vi "核查数据发送(子VI).vi"(8 "错误输入":errorcluster) -> (0 "错误输出":errorcluster)   [LabVIEW 2016, in "数据传输系统.lvlib"]
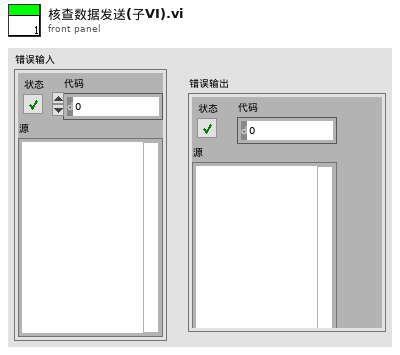
[diagram p1: front panel]
types:
  T1 = enum16{"质控数据", "操作日志", "仪器参数", "系统状态", "运行模式", "测量周期", "超标留样", "报警信息", "环境参数"}
  T2 = enum16{"空白测试", "跨度核查", "标样核查", "加标回收", "平行样", "集成干预"}
  T3 = cluster{"氨氮零点核查索引起始时间":string, "总磷零点核查索引起始时间":string, "总氮零点核查索引起始时间":string, "CODMn零点核查索引起始时间":string, "CODCr零点核查索引起始时间":string, "亚硝酸盐零点核查索引起始时间":string, "硫化物零点核查索引起始时间":string, "ORP零点核查索引起始时间":string}
  T4 = cluster{"数组[0]":string, "数组[1]":string, "数组[2]":string, "数组[3]":string, "数组[4]":string, "数组[5]":string, "数组[6]":string, "数组[7]":string}
  T5 = cluster{"PH":string[][], "CODCr":string[][], "氨氮":string[][], "CODMn":string[][], "总氮":string[][], "总磷":string[][], "电导率":string[][], "水温":string[][], "DO":string[][], "浊度":string[][], "叶绿素":string[][], "藻密度":string[][], "铜":string[][], "盐度":string[][], "水位":string[][], "流速":string[][], "瞬时流量":string[][], "累积流量":string[][], "亚硝酸盐":string[][], "硫化物":string[][], "ORP":string[][], "铅":string[][], "镉":string[][], "锌":string[][], "镍":string[][], "锰":string[][], "汞":string[][], "气温":string[][], "气压":string[][], "风速":string[][], "风向":string[][]}
  T6 = cluster{"氨氮跨度核查索引起始时间":string, "总磷跨度核查索引起始时间":string, "总氮跨度核查索引起始时间":string, "CODMn跨度核查索引起始时间":string, "CODCr跨度核查索引起始时间":string, "亚硝酸盐跨度核查索引起始时间":string, "硫化物跨度核查索引起始时间":string, "ORP跨度核查索引起始时间":string}
  T7 = cluster{"氨氮标样核查索引起始时间":string, "总磷标样核查索引起始时间":string, "总氮标样核查索引起始时间":string, "CODMn标样核查索引起始时间":string, "CODCr标样核查索引起始时间":string, "DO标样核查索引起始时间":string, "PH标样核查索引起始时间":string, "比电导率标样核查索引起始时间":string, "水温标样核查索引起始时间":string, "浊度标样核查索引起始时间":string, "叶绿素a标样核查索引起始时间":string, "藻密度标样核查索引起始时间":string, "亚硝酸盐标样核查索引起始时间":string, "硫化物标样核查索引起始时间":string, "ORP标样核查索引起始时间":string}
  T8 = cluster{"数组[0]":string, "数组[1]":string, "数组[2]":string, "数组[3]":string, "数组[4]":string, "数组[5]":string, "数组[6]":string, "数组[7]":string, "数组[8]":string, "数组[9]":string, "数组[10]":string, "数组[11]":string, "数组[12]":string, "数组[13]":string, "数组[14]":string}
  T9 = cluster{"氨氮加标回收索引起始时间":string, "总磷加标回收索引起始时间":string, "总氮加标回收索引起始时间":string, "CODMn加标回收索引起始时间":string, "CODCr加标回收索引起始时间":string}
  T10 = cluster{"[0]":string, "[1]":string, "[2]":string, "[3]":string, "[4]":string}
  T11 = cluster{"氨氮平行样索引起始时间":string, "总磷平行样索引起始时间":string, "总氮平行样索引起始时间":string, "CODMn平行样索引起始时间":string, "CODCr平行样索引起始时间":string}
  T12 = cluster{"氨氮集成干预索引起始时间":string, "总磷集成干预索引起始时间":string, "总氮集成干预索引起始时间":string, "CODMn集成干预索引起始时间":string, "CODCr集成干预索引起始时间":string, "DO集成干预索引起始时间":string, "PH集成干预索引起始时间":string, "比电导率集成干预索引起始时间":string, "水温集成干预索引起始时间":string, "浊度集成干预索引起始时间":string, "叶绿素a集成干预索引起始时间":string, "藻密度集成干预索引起始时间":string, "亚硝酸盐集成干预索引起始时间":string, "硫化物集成干预索引起始时间":string, "ORP集成干预索引起始时间":string}
  T13 = cluster{"[0]":string, "[1]":string, "[2]":string, "[3]":string, "[4]":string, "[5]":string, "[6]":string, "[7]":string, "[8]":string, "[9]":string, "[10]":string, "[11]":string, "[12]":string, "[13]":string, "[14]":string}
  T14 = cluster{"氨氮仪器日志索引起始时间":string, "总磷仪器日志索引起始时间":string, "总氮仪器日志索引起始时间":string, "CODMn仪器日志索引起始时间":string, "CODCr仪器日志索引起始时间":string, "系统仪器日志索引起始时间":string}
  T15 = cluster{"[0]":string, "[1]":string, "[2]":string, "[3]":string, "[4]":string, "[5]":string}
  T16 = cluster{"氨氮仪器参数索引起始时间":string, "总磷仪器参数索引起始时间":string, "总氮仪器参数索引起始时间":string, "CODMn仪器参数索引起始时间":string, "CODCr仪器参数索引起始时间":string, "DO仪器参数索引起始时间":string, "PH仪器参数索引起始时间":string, "比电导率仪器参数索引起始时间":string, "水温仪器参数索引起始时间":string, "浊度仪器参数索引起始时间":string, "叶绿素a仪器参数索引起始时间":string, "藻密度仪器参数索引起始时间":string, "ORP仪器参数索引起始时间":string}
  T17 = cluster{"[0]":string, "[1]":string, "[2]":string, "[3]":string, "[4]":string, "[5]":string, "[6]":string, "[7]":string, "[8]":string, "[9]":string, "[10]":string, "[11]":string, "[12]":string}
  T18 = cluster{"氨氮报警信息索引起始时间":string, "总磷报警信息索引起始时间":string, "总氮报警信息索引起始时间":string, "CODMn报警信息索引起始时间":string, "CODCr报警信息索引起始时间":string, "DO报警信息索引起始时间":string, "PH报警信息索引起始时间":string, "比电导率报警信息索引起始时间":string, "水温报警信息索引起始时间":string, "浊度报警信息索引起始时间":string, "叶绿素报警信息索引起始时间":string, "系统报警信息索引起始时间":string}
  T19 = cluster{"[0]":string, "[1]":string, "[2]":string, "[3]":string, "[4]":string, "[5]":string, "[6]":string, "[7]":string, "[8]":string, "[9]":string, "[10]":string, "[11]":string}
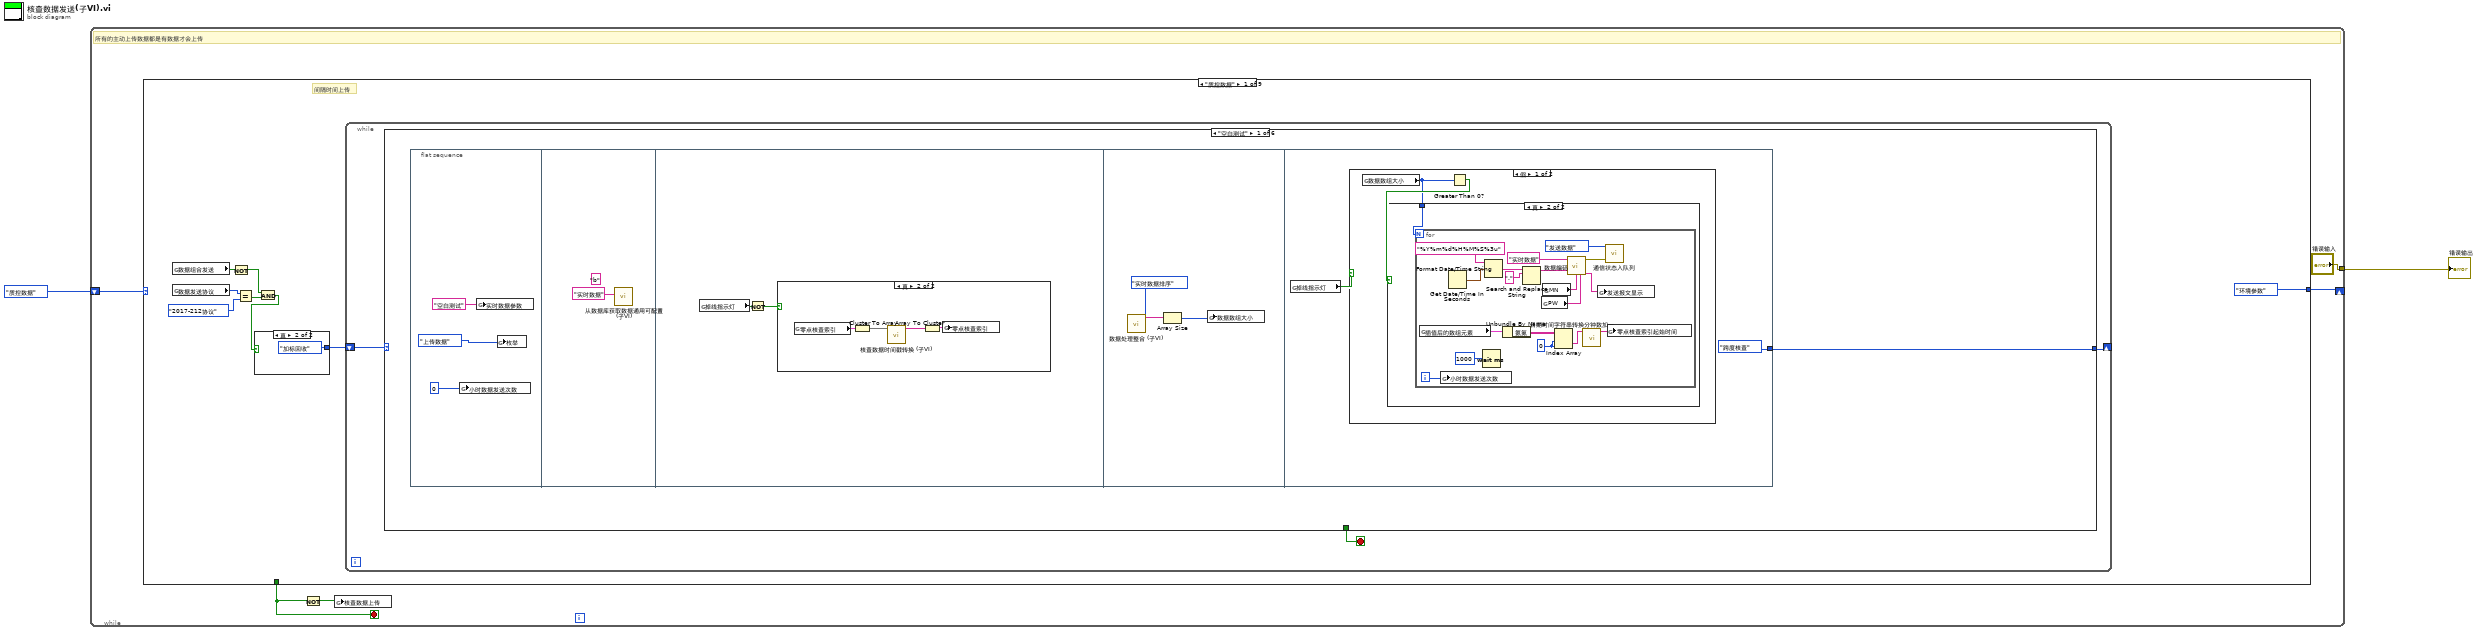
[diagram p0: block diagram]
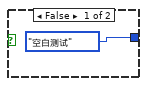
[diagram p2: hidden frame]
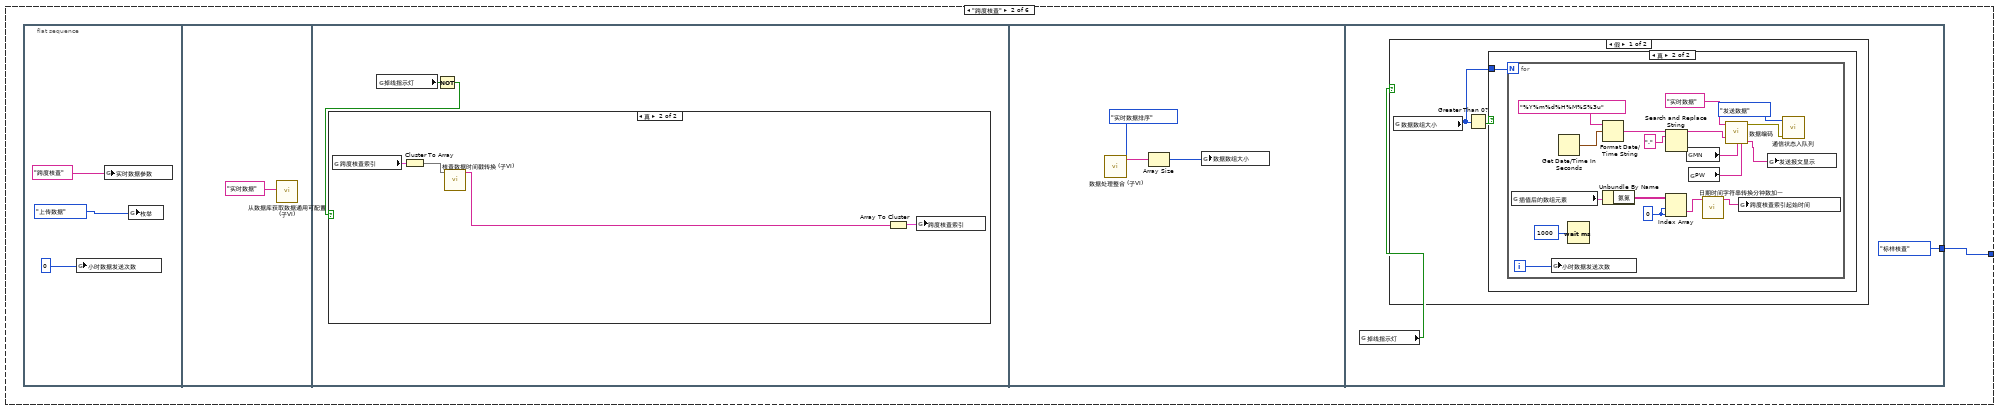
[diagram p6: hidden frame]
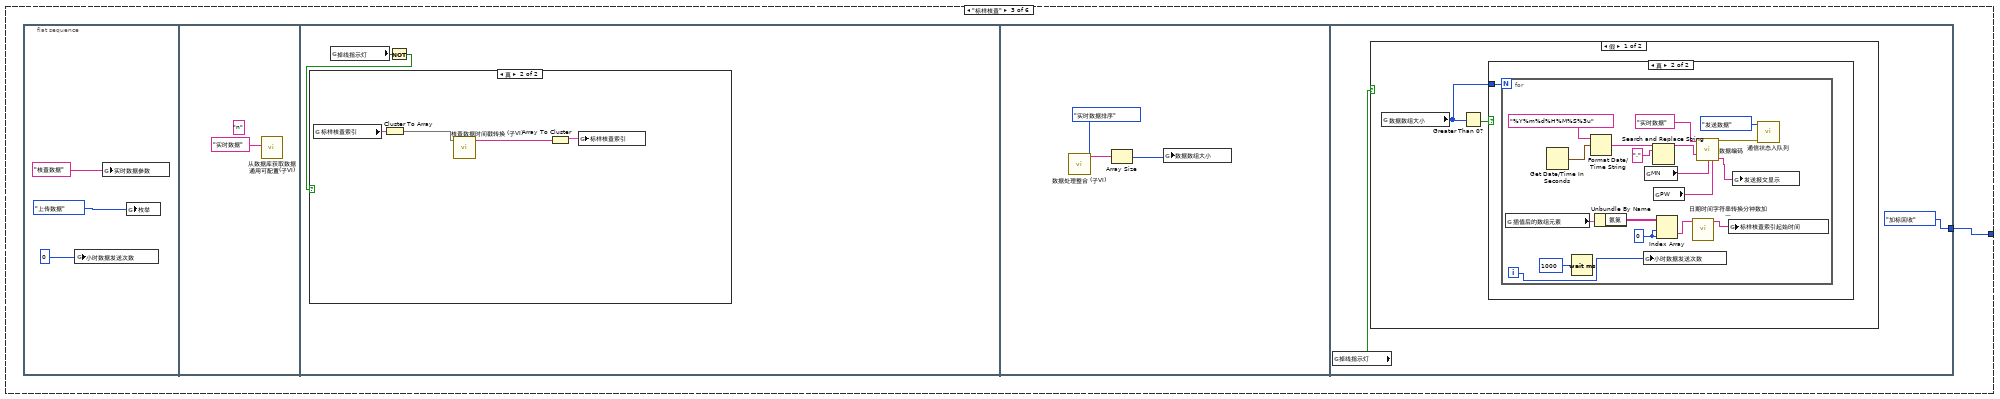
[diagram p10: hidden frame]
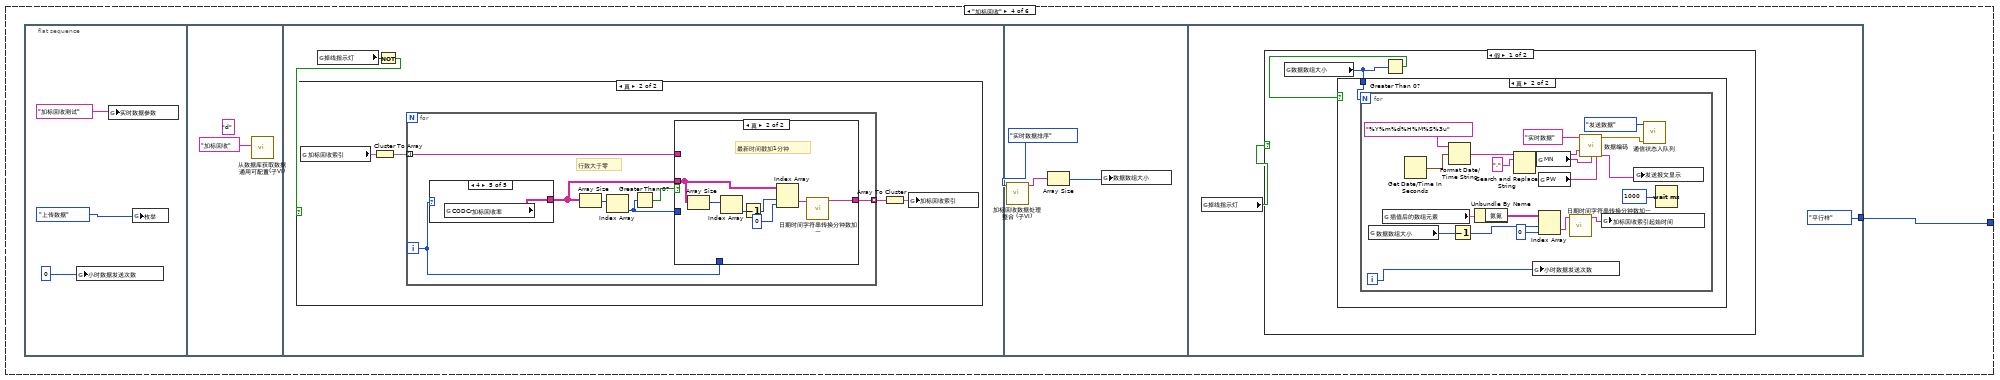
[diagram p14: hidden frame]
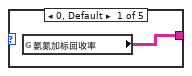
[diagram p16: hidden frame]
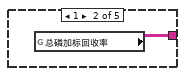
[diagram p17: hidden frame]
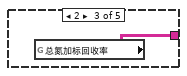
[diagram p18: hidden frame]
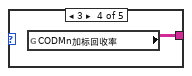
[diagram p19: hidden frame]
diagram:
  n1 = while "While循环" {
    shift-right: [w6] -> _
    shift-left: T1."质控数据" -> [w7]
    tunnel: ["错误输入"] -> w1
    stop <- w4 stop-if-true
    # "所有的主动上传数据都是有数据才会上传"
    n2 = case shown="\"质控数据\"" w7 {
      tunnel: [T1."环境参数" T1."仪器参数" T1."系统状态" T1."运行模式" T1."测量周期" T1."超标留样" T1."报警信息" T1."环境参数" T1."环境参数"] -> w6
      tunnel: [_ _ _ _ _ _ _ _ TRUE] -> w4
      frame "质控数据" {
        # "间隔时间上传"
        n3 = global read "断电保存全局.vi" "数据组合发送"() -> (w10:bool)
        n4 = global read "断电保存全局.vi" "数据发送协议"() -> (w13:enum16{"2005-212协议", "2017-212协议"})
        n5 = Not(x=w10) -> (.not. x?=w9:bool)
        n6 = Equal?(x=w13, y=enum16{"2005-212协议", "2017-212协议"}."2017-212协议" ("数据发送协议")) -> (x = y?=w11:bool)
        n7 = And(x=w9, y=w11) -> (x .and. y?=w8:bool)
        n8 = case shown="真" w8 {
          tunnel: [T2."空白测试" T2."加标回收"] -> w15
          frame False {
          }
          frame True {
          }
        }
        n9 = while {
          shift-right: [w18] -> _
          shift-left: w15 -> [w19]
          stop <- w20 stop-if-true
          n10 = case shown="\"空白测试\"" w19 {
            tunnel: [_ _ _ _ _ TRUE] -> w20
            tunnel: [w21 w58 w95 w132 w191 w243] -> w18
            frame "空白测试" {
              n11 = flat-sequence {
                tunnel: [T2."跨度核查"] -> w21
                frame #0 {
                  n12 = global write "全局 小时数据发送次数.vi" "小时数据发送次数"(0 ("小时数据发送次数")) -> ()
                  n13 = global write "全局 实时数据参数.vi" "实时数据参数"("空白测试") -> ()
                  n14 = global write "全局1.vi" "枚举"(enum16{"返回请求应答", "上传数据", "返回执行结果"}."上传数据" ("枚举")) -> ()
                }
                frame #1 {
                  (unwired) "b" ("列队名（唯一）")
                  n15 = call "从数据库获取数据通用可配置(子VI).vi"("table输入"="实时数据" ("新元素/子数组")) -> ()  [unwired: 9 in, 2 out]
                }
                frame #2 {
                  n16 = global read "全局 数据发送重叠.vi" "掉线指示灯"() -> (w27:bool)
                  n17 = Not(x=w27) -> (.not. x?=w26:bool)
                  n18 = case shown="真" w26 {
                    frame False {
                    }
                    frame True {
                      n19 = global read "全局 时间2.vi" "零点核查索引"() -> (w28:T3)
                      n20 = Cluster To Array(cluster=w28) -> (array=w31:string[])
                      n21 = call "核查数据时间戳转换 (子VI).vi"("核查索引"=w31) -> ("数组"=w30:string[])  [unwired: 10 in]
                      n22 = Array To Cluster(array=w30) -> (cluster=w29:T4)
                      n23 = global write "全局 时间2.vi" "零点核查索引"(w29) -> ()
                    }
                  }
                }
                frame #3 {
                  n24 = call "数据处理整合 (子VI).vi"("枚举"=enum16{"实时数据排序", "小时数据排序"}."实时数据排序") -> ("已排序的数组"=w34:string[])  [unwired: 10 in]
                  n25 = Array Size(array=w34) -> (size(s)=w33:i32)
                  n26 = global write "全局 数据数组大小.vi" "数据数组大小"(w33) -> ()
                }
                frame #4 {
                  n27 = global read "全局 数据发送重叠.vi" "掉线指示灯"() -> (w36:bool)
                  n28 = case shown="假" w36 {
                    frame False {
                      n29 = global read "全局 数据数组大小.vi" "数据数组大小"() -> (w37:i32)
                      n30 = Greater Than 0?(x=w37) -> (x > 0?=w38:bool)
                      n31 = case shown="真" w38 {
                        tunnel: w37 -> [_ w39]
                        frame False {
                        }
                        frame True {
                          n32 = for {
                            N: w39 -> [_]
                            i -> [w40]
                            w52 = 0 ("禁用的索引 (列)")
                            n33 = global read "插值后的新数组.vi" "插值后的数组元素"() -> (w56:T5)
                            n34 = global write "全局 小时数据发送次数.vi" "小时数据发送次数"(w40) -> ()
                            n35 = Get Date/Time In Seconds() -> (seconds since 1Jan1904=w44:timestamp)
                            n36 = Wait (ms)(milliseconds to wait=u32 1000 ("等待时间（毫秒）")) -> ()  [unwired: 1 out]
                            n37 = Format Date/Time String(time format string (%c)="%Y%m%d%H%M%S%3u" ("时间格式字符串(%c)"), seconds (now)=w44) -> (date/time string=w43:string)  [unwired: 1 in]
                            n38 = Unbundle By Name(w56) -> ("氨氮"=w55:string[][])
                            n39 = Search and Replace String(input string=w43, search string="." ("搜索字符串")) -> (result string=w41:string)  [unwired: 6 in, 3 out]
                            n40 = global read "断电保存全局.vi" "PW"() -> (w48:string)
                            n41 = global read "断电保存全局.vi" "MN"() -> (w49:string)
                            n42 = Index Array(array=w55, index (row)=w52, index (col)=w52) -> (element=w54:string)
                            n43 = call "数据编码.vi"("table输入"="实时数据" ("新元素/子数组"), "QN"=w41, "MN"=w49, "PW"=w48) -> ("错误常量"=w47:errorcluster, "通讯包字符串"=w51:string)  [unwired: 10 in]
                            n44 = call "日期时间字符串转换分钟数加一.vi"("data[0]"=w54) -> ("日期/时间字符串"=w53:string)  [unwired: 10 in]
                            n45 = global write "全局1.vi" "发送报文显示"(w51) -> ()
                            n46 = call "通信状态入队列.vi"("错误输入（无错误）"=w47, "枚举"=enum16{"打开连接", "发送数据", "读取数据", "数据处理", "关闭连接"}."发送数据") -> ()  [unwired: 9 in, 1 out]
                            n47 = global write "全局 时间2.vi" "零点核查索引起始时间"(w53) -> ()
                          }
                        }
                      }
                    }
                    frame True {
                    }
                  }
                }
              }
            }
            frame "跨度核查" {
              n48 = flat-sequence {
                tunnel: [T2."标样核查"] -> w58
                frame #0 {
                  n49 = global write "全局 小时数据发送次数.vi" "小时数据发送次数"(0 ("小时数据发送次数")) -> ()
                  n50 = global write "全局 实时数据参数.vi" "实时数据参数"("跨度核查") -> ()
                  n51 = global write "全局1.vi" "枚举"(enum16{"返回请求应答", "上传数据", "返回执行结果"}."上传数据" ("枚举")) -> ()
                }
                frame #1 {
                  n52 = call "从数据库获取数据通用可配置(子VI).vi"("table输入"="实时数据" ("新元素/子数组")) -> ()  [unwired: 9 in, 2 out]
                }
                frame #2 {
                  n53 = global read "全局 数据发送重叠.vi" "掉线指示灯"() -> (w64:bool)
                  n54 = Not(x=w64) -> (.not. x?=w63:bool)
                  n55 = case shown="真" w63 {
                    frame False {
                    }
                    frame True {
                      n56 = global read "全局 时间2.vi" "跨度核查索引"() -> (w68:T6)
                      n57 = Cluster To Array(cluster=w68) -> (array=w66:string[])
                      n58 = call "核查数据时间戳转换 (子VI).vi"("核查索引"=w66) -> ("数组"=w65:string[])  [unwired: 10 in]
                      n59 = Array To Cluster(array=w65) -> (cluster=w67:T4)
                      n60 = global write "全局 时间2.vi" "跨度核查索引"(w67) -> ()
                    }
                  }
                }
                frame #3 {
                  n61 = call "数据处理整合 (子VI).vi"("枚举"=enum16{"实时数据排序", "小时数据排序"}."实时数据排序") -> ("已排序的数组"=w71:string[])  [unwired: 10 in]
                  n62 = Array Size(array=w71) -> (size(s)=w70:i32)
                  n63 = global write "全局 数据数组大小.vi" "数据数组大小"(w70) -> ()
                }
                frame #4 {
                  n64 = global read "全局 数据发送重叠.vi" "掉线指示灯"() -> (w73:bool)
                  n65 = case shown="假" w73 {
                    frame False {
                      n66 = global read "全局 数据数组大小.vi" "数据数组大小"() -> (w74:i32)
                      n67 = Greater Than 0?(x=w74) -> (x > 0?=w75:bool)
                      n68 = case shown="真" w75 {
                        tunnel: w74 -> [_ w76]
                        frame False {
                        }
                        frame True {
                          n69 = for {
                            N: w76 -> [_]
                            i -> [w77]
                            w89 = 0 ("禁用的索引 (列)")
                            n70 = global read "插值后的新数组.vi" "插值后的数组元素"() -> (w93:T5)
                            n71 = global write "全局 小时数据发送次数.vi" "小时数据发送次数"(w77) -> ()
                            n72 = Get Date/Time In Seconds() -> (seconds since 1Jan1904=w81:timestamp)
                            n73 = Wait (ms)(milliseconds to wait=u32 1000 ("等待时间（毫秒）")) -> ()  [unwired: 1 out]
                            n74 = Format Date/Time String(time format string (%c)="%Y%m%d%H%M%S%3u" ("时间格式字符串(%c)"), seconds (now)=w81) -> (date/time string=w80:string)  [unwired: 1 in]
                            n75 = Unbundle By Name(w93) -> ("氨氮"=w92:string[][])
                            n76 = Index Array(array=w92, index (row)=w89, index (col)=w89) -> (element=w91:string)
                            n77 = Search and Replace String(input string=w80, search string="." ("搜索字符串")) -> (result string=w78:string)  [unwired: 6 in, 3 out]
                            n78 = global read "断电保存全局.vi" "MN"() -> (w87:string)
                            n79 = global read "断电保存全局.vi" "PW"() -> (w86:string)
                            n80 = call "日期时间字符串转换分钟数加一.vi"("data[0]"=w91) -> ("日期/时间字符串"=w90:string)  [unwired: 10 in]
                            n81 = call "数据编码.vi"("table输入"="实时数据" ("新元素/子数组"), "QN"=w78, "MN"=w87, "PW"=w86) -> ("错误常量"=w84:errorcluster, "通讯包字符串"=w85:string)  [unwired: 10 in]
                            n82 = global write "全局 时间2.vi" "跨度核查索引起始时间"(w90) -> ()
                            n83 = global write "全局1.vi" "发送报文显示"(w85) -> ()
                            n84 = call "通信状态入队列.vi"("错误输入（无错误）"=w84, "枚举"=enum16{"打开连接", "发送数据", "读取数据", "数据处理", "关闭连接"}."发送数据") -> ()  [unwired: 9 in, 1 out]
                          }
                        }
                      }
                    }
                    frame True {
                    }
                  }
                }
              }
            }
            frame "标样核查" {
              n85 = flat-sequence {
                tunnel: [T2."加标回收"] -> w95
                frame #0 {
                  n86 = global write "全局 小时数据发送次数.vi" "小时数据发送次数"(0 ("小时数据发送次数")) -> ()
                  n87 = global write "全局 实时数据参数.vi" "实时数据参数"("核查数据") -> ()
                  n88 = global write "全局1.vi" "枚举"(enum16{"返回请求应答", "上传数据", "返回执行结果"}."上传数据" ("枚举")) -> ()
                }
                frame #1 {
                  (unwired) "n" ("列队名（唯一）")
                  n89 = call "从数据库获取数据通用可配置(子VI).vi"("table输入"="实时数据" ("新元素/子数组")) -> ()  [unwired: 9 in, 2 out]
                }
                frame #2 {
                  n90 = global read "全局 数据发送重叠.vi" "掉线指示灯"() -> (w101:bool)
                  n91 = Not(x=w101) -> (.not. x?=w100:bool)
                  n92 = case shown="真" w100 {
                    frame False {
                    }
                    frame True {
                      n93 = global read "全局 时间2.vi" "标样核查索引"() -> (w105:T7)
                      n94 = Cluster To Array(cluster=w105) -> (array=w103:string[])
                      n95 = call "核查数据时间戳转换 (子VI).vi"("核查索引"=w103) -> ("数组"=w102:string[])  [unwired: 10 in]
                      n96 = Array To Cluster(array=w102) -> (cluster=w104:T8)
                      n97 = global write "全局 时间2.vi" "标样核查索引"(w104) -> ()
                    }
                  }
                }
                frame #3 {
                  n98 = call "数据处理整合 (子VI).vi"("枚举"=enum16{"实时数据排序", "小时数据排序"}."实时数据排序") -> ("已排序的数组"=w108:string[])  [unwired: 10 in]
                  n99 = Array Size(array=w108) -> (size(s)=w107:i32)
                  n100 = global write "全局 数据数组大小.vi" "数据数组大小"(w107) -> ()
                }
                frame #4 {
                  n101 = global read "全局 数据发送重叠.vi" "掉线指示灯"() -> (w110:bool)
                  n102 = case shown="假" w110 {
                    frame False {
                      n103 = global read "全局 数据数组大小.vi" "数据数组大小"() -> (w111:i32)
                      n104 = Greater Than 0?(x=w111) -> (x > 0?=w112:bool)
                      n105 = case shown="真" w112 {
                        tunnel: w111 -> [_ w113]
                        frame False {
                        }
                        frame True {
                          n106 = for {
                            N: w113 -> [_]
                            i -> [w114]
                            w126 = 0 ("禁用的索引 (列)")
                            n107 = global read "插值后的新数组.vi" "插值后的数组元素"() -> (w130:T5)
                            n108 = Get Date/Time In Seconds() -> (seconds since 1Jan1904=w118:timestamp)
                            n109 = Wait (ms)(milliseconds to wait=u32 1000 ("等待时间（毫秒）")) -> ()  [unwired: 1 out]
                            n110 = Format Date/Time String(time format string (%c)="%Y%m%d%H%M%S%3u" ("时间格式字符串(%c)"), seconds (now)=w118) -> (date/time string=w117:string)  [unwired: 1 in]
                            n111 = Unbundle By Name(w130) -> ("氨氮"=w129:string[][])
                            n112 = global write "全局 小时数据发送次数.vi" "小时数据发送次数"(w114) -> ()
                            n113 = global read "断电保存全局.vi" "MN"() -> (w123:string)
                            n114 = Search and Replace String(input string=w117, search string="." ("搜索字符串")) -> (result string=w115:string)  [unwired: 6 in, 3 out]
                            n115 = global read "断电保存全局.vi" "PW"() -> (w122:string)
                            n116 = Index Array(array=w129, index (row)=w126, index (col)=w126) -> (element=w128:string)
                            n117 = call "日期时间字符串转换分钟数加一.vi"("data[0]"=w128) -> ("日期/时间字符串"=w127:string)  [unwired: 10 in]
                            n118 = call "数据编码.vi"("table输入"="实时数据" ("新元素/子数组"), "QN"=w115, "MN"=w123, "PW"=w122) -> ("错误常量"=w121:errorcluster, "通讯包字符串"=w125:string)  [unwired: 10 in]
                            n119 = global write "全局 时间2.vi" "标样核查索引起始时间"(w127) -> ()
                            n120 = global write "全局1.vi" "发送报文显示"(w125) -> ()
                            n121 = call "通信状态入队列.vi"("错误输入（无错误）"=w121, "枚举"=enum16{"打开连接", "发送数据", "读取数据", "数据处理", "关闭连接"}."发送数据") -> ()  [unwired: 9 in, 1 out]
                          }
                        }
                      }
                    }
                    frame True {
                    }
                  }
                }
              }
            }
            frame "加标回收" {
              n122 = flat-sequence {
                tunnel: [T2."平行样"] -> w132
                frame #0 {
                  n123 = global write "全局 小时数据发送次数.vi" "小时数据发送次数"(0 ("小时数据发送次数")) -> ()
                  n124 = global write "全局 实时数据参数.vi" "实时数据参数"("加标回收测试") -> ()
                  n125 = global write "全局1.vi" "枚举"(enum16{"返回请求应答", "上传数据", "返回执行结果"}."上传数据" ("枚举")) -> ()
                }
                frame #1 {
                  (unwired) "d" ("列队名（唯一）")
                  n126 = call "从数据库获取数据通用可配置(子VI).vi"("table输入"="加标回收" ("新元素/子数组")) -> ()  [unwired: 9 in, 2 out]
                }
                frame #2 {
                  n127 = global read "全局 数据发送重叠.vi" "掉线指示灯"() -> (w138:bool)
                  n128 = Not(x=w138) -> (.not. x?=w137:bool)
                  n129 = case shown="真" w137 {
                    frame False {
                    }
                    frame True {
                      n130 = global read "全局 时间2.vi" "加标回收索引"() -> (w142:T9)
                      n131 = Cluster To Array(cluster=w142) -> (array=w141:string[])
                      n132 = for {
                        tunnel: [w144] -> w139 mode=indexing
                        tunnel: w141 -> [w143] mode=indexing
                        i -> [w145]
                        # "行数大于零"
                        n133 = case shown="4" w145 {
                          tunnel: [w150 w151 w152 w153 w154] -> w146
                          frame 0, Default {
                            n134 = global read "全局 所有参数.vi" "氨氮加标回收率"() -> (w150:string[][])
                          }
                          frame 1 {
                            n135 = global read "全局 所有参数.vi" "总磷加标回收率"() -> (w151:string[][])
                          }
                          frame 2 {
                            n136 = global read "全局 所有参数.vi" "总氮加标回收率"() -> (w152:string[][])
                          }
                          frame 3 {
                            n137 = global read "全局 所有参数.vi" "CODMn加标回收率"() -> (w153:string[][])
                          }
                          frame 4 {
                            n138 = global read "全局 所有参数.vi" "CODCr加标回收率"() -> (w154:string[][])
                          }
                        }
                        n139 = Array Size(array=w146) -> (size(s)=w148:i32[])
                        n140 = Index Array(array=w148) -> (element=w147:i32)  [unwired: 1 in]
                        n141 = Greater Than 0?(x=w147) -> (x > 0?=w149:bool)
                        n142 = case shown="真" w149 {
                          tunnel: w145 -> [_ _]
                          tunnel: w147 -> [_ _]
                          tunnel: w146 -> [_ w159]
                          tunnel: [w155 w156] -> w144
                          tunnel: w143 -> [w155 _]
                          frame False {
                          }
                          frame True {
                            # "最新时间戳加1分钟"
                            n143 = Array Size(array=w159) -> (size(s)=w161:i32[])
                            n144 = Index Array(array=w161) -> (element=w160:i32)  [unwired: 1 in]
                            n145 = Decrement(x=w160) -> (x-1=w158:i32)
                            n146 = Index Array(array=w159, index (row)=w158, index (col)=0 ("禁用的索引 (列)")) -> (element=w162:string)
                            n147 = call "日期时间字符串转换分钟数加一.vi"("data[0]"=w162) -> ("日期/时间字符串"=w156:string)  [unwired: 10 in]
                          }
                        }
                      }
                      n148 = Array To Cluster(array=w139) -> (cluster=w140:T10)
                      n149 = global write "全局 时间2.vi" "加标回收索引"(w140) -> ()
                    }
                  }
                }
                frame #3 {
                  n150 = call "加标回收数据处理整合 (子VI).vi"("枚举"=enum16{"实时数据排序", "小时数据排序"}."实时数据排序") -> ("已排序的数组"=w164:string[])  [unwired: 10 in]
                  n151 = Array Size(array=w164) -> (size(s)=w165:i32)
                  n152 = global write "全局 数据数组大小.vi" "数据数组大小"(w165) -> ()
                }
                frame #4 {
                  n153 = global read "全局 数据发送重叠.vi" "掉线指示灯"() -> (w167:bool)
                  n154 = case shown="假" w167 {
                    frame False {
                      n155 = global read "全局 数据数组大小.vi" "数据数组大小"() -> (w168:i32)
                      n156 = Greater Than 0?(x=w168) -> (x > 0?=w169:bool)
                      n157 = case shown="真" w169 {
                        tunnel: w168 -> [_ w170]
                        frame False {
                        }
                        frame True {
                          n158 = for {
                            N: w170 -> [_]
                            i -> [w171]
                            n159 = global read "全局 数据数组大小.vi" "数据数组大小"() -> (w186:i32)
                            n160 = global read "插值后的新数组.vi" "插值后的数组元素"() -> (w189:T5)
                            n161 = Get Date/Time In Seconds() -> (seconds since 1Jan1904=w175:timestamp)
                            n162 = Format Date/Time String(time format string (%c)="%Y%m%d%H%M%S%3u" ("时间格式字符串(%c)"), seconds (now)=w175) -> (date/time string=w174:string)  [unwired: 1 in]
                            n163 = Decrement(x=w186) -> (x-1=w185:i32)
                            n164 = Unbundle By Name(w189) -> ("氨氮"=w188:string[][])
                            n165 = Search and Replace String(input string=w174, search string="." ("搜索字符串")) -> (result string=w172:string)  [unwired: 6 in, 3 out]
                            n166 = global write "全局 小时数据发送次数.vi" "小时数据发送次数"(w171) -> ()
                            n167 = global read "断电保存全局.vi" "MN"() -> (w180:string)
                            n168 = Index Array(array=w188, index (row)=w185, index (col)=0 ("禁用的索引 (列)")) -> (element=w184:string)
                            n169 = global read "断电保存全局.vi" "PW"() -> (w179:string)
                            n170 = call "日期时间字符串转换分钟数加一.vi"("data[0]"=w184) -> ("日期/时间字符串"=w183:string)  [unwired: 10 in]
                            n171 = call "数据编码.vi"("table输入"="实时数据" ("新元素/子数组"), "QN"=w172, "MN"=w180, "PW"=w179) -> ("错误常量"=w178:errorcluster, "通讯包字符串"=w182:string)  [unwired: 10 in]
                            n172 = global write "全局 时间2.vi" "加标回收索引起始时间"(w183) -> ()
                            n173 = global write "全局1.vi" "发送报文显示"(w182) -> ()
                            n174 = call "通信状态入队列.vi"("错误输入（无错误）"=w178, "枚举"=enum16{"打开连接", "发送数据", "读取数据", "数据处理", "关闭连接"}."发送数据") -> ()  [unwired: 9 in, 1 out]
                            n175 = Wait (ms)(milliseconds to wait=u32 1000 ("等待时间（毫秒）")) -> ()  [unwired: 1 out]
                          }
                        }
                      }
                    }
                    frame True {
                    }
                  }
                }
              }
            }
            frame "平行样" {
              n176 = flat-sequence {
                tunnel: [T2."集成干预"] -> w191
                frame #0 {
                  n177 = global write "全局 小时数据发送次数.vi" "小时数据发送次数"(0 ("小时数据发送次数")) -> ()
                  n178 = global write "全局 实时数据参数.vi" "实时数据参数"("平行样测试") -> ()
                  n179 = global write "全局1.vi" "枚举"(enum16{"返回请求应答", "上传数据", "返回执行结果"}."上传数据" ("枚举")) -> ()
                }
                frame #1 {
                  (unwired) "e" ("列队名（唯一）")
                  n180 = call "从数据库获取数据通用可配置(子VI).vi"("table输入"="平行样测试" ("新元素/子数组")) -> ()  [unwired: 9 in, 2 out]
                }
                frame #2 {
                  n181 = global read "全局 数据发送重叠.vi" "掉线指示灯"() -> (w197:bool)
                  n182 = Not(x=w197) -> (.not. x?=w196:bool)
                  n183 = case shown="真" w196 {
                    frame False {
                    }
                    frame True {
                      n184 = global read "全局 时间2.vi" "平行样索引"() -> (w201:T11)
                      n185 = Cluster To Array(cluster=w201) -> (array=w200:string[])
                      n186 = for {
                        tunnel: [w203] -> w198 mode=indexing
                        tunnel: w200 -> [w202] mode=indexing
                        i -> [w204]
                        # "行数大于零"
                        n187 = case shown="4" w204 {
                          tunnel: [w209 w210 w211 w212 w213] -> w205
                          frame 0, Default {
                            n188 = global read "全局 所有参数.vi" "氨氮"() -> (w209:string[][])
                          }
                          frame 1 {
                            n189 = global read "全局 所有参数.vi" "总磷"() -> (w210:string[][])
                          }
                          frame 2 {
                            n190 = global read "全局 所有参数.vi" "总氮"() -> (w211:string[][])
                          }
                          frame 3 {
                            n191 = global read "全局 所有参数.vi" "CODMn"() -> (w212:string[][])
                          }
                          frame 4 {
                            n192 = global read "全局 所有参数.vi" "CODCr"() -> (w213:string[][])
                          }
                        }
                        n193 = Array Size(array=w205) -> (size(s)=w207:i32[])
                        n194 = Index Array(array=w207) -> (element=w206:i32)  [unwired: 1 in]
                        n195 = Greater Than 0?(x=w206) -> (x > 0?=w208:bool)
                        n196 = case shown="真" w208 {
                          tunnel: w204 -> [_ _]
                          tunnel: w206 -> [_ _]
                          tunnel: w205 -> [_ w218]
                          tunnel: [w214 w215] -> w203
                          tunnel: w202 -> [w214 _]
                          frame False {
                          }
                          frame True {
                            # "最新时间戳加1分钟"
                            n197 = Array Size(array=w218) -> (size(s)=w220:i32[])
                            n198 = Index Array(array=w220) -> (element=w219:i32)  [unwired: 1 in]
                            n199 = Decrement(x=w219) -> (x-1=w217:i32)
                            n200 = Index Array(array=w218, index (row)=w217, index (col)=0 ("禁用的索引 (列)")) -> (element=w221:string)
                            n201 = call "日期时间字符串转换分钟数加一.vi"("data[0]"=w221) -> ("日期/时间字符串"=w215:string)  [unwired: 10 in]
                          }
                        }
                      }
                      n202 = Array To Cluster(array=w198) -> (cluster=w199:T10)
                      n203 = global write "全局 时间2.vi" "平行样索引"(w199) -> ()
                    }
                  }
                }
                frame #3 {
                  n204 = call "数据处理整合 (子VI).vi"("枚举"=enum16{"实时数据排序", "小时数据排序"}."实时数据排序") -> ("已排序的数组"=w224:string[])  [unwired: 10 in]
                  n205 = Array Size(array=w224) -> (size(s)=w223:i32)
                  n206 = global write "全局 数据数组大小.vi" "数据数组大小"(w223) -> ()
                }
                frame #4 {
                  n207 = global read "全局 数据发送重叠.vi" "掉线指示灯"() -> (w225:bool)
                  n208 = case shown="假" w225 {
                    frame False {
                      n209 = global read "全局 数据数组大小.vi" "数据数组大小"() -> (w227:i32)
                      n210 = Greater Than 0?(x=w227) -> (x > 0?=w228:bool)
                      n211 = case shown="真" w228 {
                        tunnel: w227 -> [_ w229]
                        frame False {
                        }
                        frame True {
                          n212 = for {
                            N: w229 -> [_]
                            i -> [w230]
                            n213 = Get Date/Time In Seconds() -> (seconds since 1Jan1904=w234:timestamp)
                            n214 = global write "全局 小时数据发送次数.vi" "小时数据发送次数"(w230) -> ()
                            n215 = Format Date/Time String(time format string (%c)="%Y%m%d%H%M%S%3u" ("时间格式字符串(%c)"), seconds (now)=w234) -> (date/time string=w233:string)  [unwired: 1 in]
                            n216 = Search and Replace String(input string=w233, search string="." ("搜索字符串")) -> (result string=w231:string)  [unwired: 6 in, 3 out]
                            n217 = global read "断电保存全局.vi" "MN"() -> (w239:string)
                            n218 = global read "断电保存全局.vi" "PW"() -> (w238:string)
                            n219 = call "数据编码.vi"("table输入"="实时数据" ("新元素/子数组"), "QN"=w231, "MN"=w239, "PW"=w238) -> ("错误常量"=w237:errorcluster, "通讯包字符串"=w241:string)  [unwired: 10 in]
                            n220 = global write "全局1.vi" "发送报文显示"(w241) -> ()
                            n221 = call "通信状态入队列.vi"("错误输入（无错误）"=w237, "枚举"=enum16{"打开连接", "发送数据", "读取数据", "数据处理", "关闭连接"}."发送数据") -> ()  [unwired: 9 in, 1 out]
                            n222 = Wait (ms)(milliseconds to wait=u32 1000 ("等待时间（毫秒）")) -> ()  [unwired: 1 out]
                          }
                        }
                      }
                    }
                    frame True {
                    }
                  }
                }
              }
            }
            frame "集成干预" {
              n223 = flat-sequence {
                tunnel: [T2."集成干预"] -> w243
                frame #0 {
                  n224 = global write "全局 小时数据发送次数.vi" "小时数据发送次数"(0 ("小时数据发送次数")) -> ()
                  n225 = global write "全局 实时数据参数.vi" "实时数据参数"("集成干预测试") -> ()
                  n226 = global write "全局1.vi" "枚举"(enum16{"返回请求应答", "上传数据", "返回执行结果"}."上传数据" ("枚举")) -> ()
                }
                frame #1 {
                  (unwired) "f" ("列队名（唯一）")
                  n227 = call "从数据库获取数据通用可配置(子VI).vi"("table输入"="集成干预测试" ("新元素/子数组")) -> ()  [unwired: 9 in, 2 out]
                }
                frame #2 {
                  n228 = global read "全局 数据发送重叠.vi" "掉线指示灯"() -> (w250:bool)
                  n229 = Not(x=w250) -> (.not. x?=w249:bool)
                  n230 = case shown="真" w249 {
                    frame False {
                    }
                    frame True {
                      n231 = global read "全局 时间2.vi" "集成干预索引"() -> (w254:T12)
                      n232 = Cluster To Array(cluster=w254) -> (array=w253:string[])
                      n233 = for {
                        tunnel: [w256] -> w251 mode=indexing
                        tunnel: w253 -> [w255] mode=indexing
                        i -> [w257]
                        # "行数大于零"
                        n234 = case shown="0, 默认" w257 {
                          tunnel: [w262 w263 w264 w265 w266 w267 w268 w269 w270 w271 w272 w273 w274 w275 w276] -> w258
                          frame 0, Default {
                            n235 = global read "全局 所有参数.vi" "氨氮"() -> (w262:string[][])
                          }
                          frame 1 {
                            n236 = global read "全局 所有参数.vi" "总磷"() -> (w263:string[][])
                          }
                          frame 2 {
                            n237 = global read "全局 所有参数.vi" "总氮"() -> (w264:string[][])
                          }
                          frame 3 {
                            n238 = global read "全局 所有参数.vi" "CODMn"() -> (w265:string[][])
                          }
                          frame 4 {
                            n239 = global read "全局 所有参数.vi" "CODCr"() -> (w266:string[][])
                          }
                          frame 5 {
                            n240 = global read "全局 所有参数.vi" "DO"() -> (w267:string[][])
                          }
                          frame 6 {
                            n241 = global read "全局 所有参数.vi" "PH"() -> (w268:string[][])
                          }
                          frame 7 {
                            n242 = global read "全局 所有参数.vi" "电导率"() -> (w269:string[][])
                          }
                          frame 8 {
                            n243 = global read "全局 所有参数.vi" "水温"() -> (w270:string[][])
                          }
                          frame 9 {
                            n244 = global read "全局 所有参数.vi" "浊度"() -> (w271:string[][])
                          }
                          frame 10 {
                            n245 = global read "全局 所有参数.vi" "叶绿素"() -> (w272:string[][])
                          }
                          frame 11 {
                            n246 = global read "全局 所有参数.vi" "藻密度"() -> (w273:string[][])
                          }
                          frame 12 {
                            n247 = global read "全局 所有参数.vi" "亚硝酸盐"() -> (w274:string[][])
                          }
                          frame 13 {
                            n248 = global read "全局 所有参数.vi" "硫化物"() -> (w275:string[][])
                          }
                          frame 14 {
                            n249 = global read "全局 所有参数.vi" "ORP"() -> (w276:string[][])
                          }
                        }
                        n250 = Array Size(array=w258) -> (size(s)=w260:i32[])
                        n251 = Index Array(array=w260) -> (element=w259:i32)  [unwired: 1 in]
                        n252 = Greater Than 0?(x=w259) -> (x > 0?=w261:bool)
                        n253 = case shown="真" w261 {
                          tunnel: w257 -> [_ _]
                          tunnel: w259 -> [_ _]
                          tunnel: w258 -> [_ w279]
                          tunnel: [w277 w278] -> w256
                          tunnel: w255 -> [w277 _]
                          frame False {
                          }
                          frame True {
                            # "最新时间戳加1分钟"
                            n254 = Array Size(array=w279) -> (size(s)=w283:i32[])
                            n255 = Index Array(array=w283) -> (element=w282:i32)  [unwired: 1 in]
                            n256 = Decrement(x=w282) -> (x-1=w281:i32)
                            n257 = Index Array(array=w279, index (row)=w281, index (col)=0 ("禁用的索引 (列)")) -> (element=w284:string)
                            n258 = call "日期时间字符串转换分钟数加一.vi"("data[0]"=w284) -> ("日期/时间字符串"=w278:string)  [unwired: 10 in]
                          }
                        }
                      }
                      n259 = Array To Cluster(array=w251) -> (cluster=w252:T13)
                      n260 = global write "全局 时间2.vi" "集成干预索引"(w252) -> ()
                    }
                  }
                }
                frame #3 {
                  n261 = call "数据处理整合 (子VI).vi"("枚举"=enum16{"实时数据排序", "小时数据排序"}."实时数据排序") -> ("已排序的数组"=w287:string[])  [unwired: 10 in]
                  n262 = Array Size(array=w287) -> (size(s)=w286:i32)
                  n263 = global write "全局 数据数组大小.vi" "数据数组大小"(w286) -> ()
                }
                frame #4 {
                  n264 = global read "全局 数据发送重叠.vi" "掉线指示灯"() -> (w289:bool)
                  n265 = case shown="假" w289 {
                    frame False {
                      n266 = global read "全局 数据数组大小.vi" "数据数组大小"() -> (w290:i32)
                      n267 = Greater Than 0?(x=w290) -> (x > 0?=w291:bool)
                      n268 = case shown="真" w291 {
                        tunnel: w290 -> [_ w292]
                        frame False {
                        }
                        frame True {
                          n269 = for {
                            N: w292 -> [_]
                            i -> [w293]
                            n270 = Get Date/Time In Seconds() -> (seconds since 1Jan1904=w297:timestamp)
                            n271 = Format Date/Time String(time format string (%c)="%Y%m%d%H%M%S%3u" ("时间格式字符串(%c)"), seconds (now)=w297) -> (date/time string=w296:string)  [unwired: 1 in]
                            n272 = global write "全局 小时数据发送次数.vi" "小时数据发送次数"(w293) -> ()
                            n273 = global read "断电保存全局.vi" "MN"() -> (w301:string)
                            n274 = global read "断电保存全局.vi" "PW"() -> (w300:string)
                            n275 = Search and Replace String(input string=w296, search string="." ("搜索字符串")) -> (result string=w294:string)  [unwired: 6 in, 3 out]
                            n276 = call "数据编码.vi"("table输入"="实时数据" ("新元素/子数组"), "QN"=w294, "MN"=w301, "PW"=w300) -> ("错误常量"=w302:errorcluster, "通讯包字符串"=w304:string)  [unwired: 10 in]
                            n277 = global write "全局1.vi" "发送报文显示"(w304) -> ()
                            n278 = call "通信状态入队列.vi"("错误输入（无错误）"=w302, "枚举"=enum16{"打开连接", "发送数据", "读取数据", "数据处理", "关闭连接"}."发送数据") -> ()  [unwired: 9 in, 1 out]
                            n279 = Wait (ms)(milliseconds to wait=u32 1000 ("等待时间（毫秒）")) -> ()  [unwired: 1 out]
                          }
                        }
                      }
                    }
                    frame True {
                    }
                  }
                }
              }
            }
          }
        }
      }
      frame "操作日志" {
        # "间隔时间上传"
        # "直接1分钟查询 一次,有数据就按数据上传,没数据就不上传,在数据发送那边有做处理"
        n280 = flat-sequence {
          frame #0 {
            # "时间"
            n281 = global write "全局 小时数据发送次数.vi" "小时数据发送次数"(0 ("小时数据发送次数")) -> ()
            n282 = call "日志信息主动发送(子VI).vi"() -> ()  [unwired: 12 in]
            n283 = global write "全局1.vi" "枚举"(enum16{"返回请求应答", "上传数据", "返回执行结果"}."上传数据" ("枚举")) -> ()
          }
          frame #1 {
            n284 = call "获取操作日志 (子VI).vi"("table输入"="操作日志") -> ()  [unwired: 11 in]
          }
          frame #2 {
            n285 = global read "全局 数据发送重叠.vi" "掉线指示灯"() -> (w311:bool)
            n286 = Not(x=w311) -> (.not. x?=w310:bool)
            n287 = case shown="真" w310 {
              frame False {
              }
              frame True {
                n288 = global read "全局 时间2.vi" "仪器日志索引"() -> (w315:T14)
                n289 = Cluster To Array(cluster=w315) -> (array=w314:string[])
                n290 = for {
                  tunnel: w314 -> [w316] mode=indexing
                  tunnel: [w317] -> w312 mode=indexing
                  i -> [w319]
                  # "行数大于零"
                  n291 = case shown="5" w319 {
                    tunnel: [w323 w324 w325 w326 w327 w328] -> w318
                    frame 0, Default {
                      n292 = global read "全局 所有参数.vi" "氨氮"() -> (w323:string[][])
                    }
                    frame 1 {
                      n293 = global read "全局 所有参数.vi" "总磷"() -> (w324:string[][])
                    }
                    frame 2 {
                      n294 = global read "全局 所有参数.vi" "总氮"() -> (w325:string[][])
                    }
                    frame 3 {
                      n295 = global read "全局 所有参数.vi" "CODMn"() -> (w326:string[][])
                    }
                    frame 4 {
                      n296 = global read "全局 所有参数.vi" "CODCr"() -> (w327:string[][])
                    }
                    frame 5 {
                      n297 = global read "全局 所有参数.vi" "DO"() -> (w328:string[][])
                    }
                  }
                  n298 = Array Size(array=w318) -> (size(s)=w321:i32[])
                  n299 = Index Array(array=w321) -> (element=w320:i32)  [unwired: 1 in]
                  n300 = Greater Than 0?(x=w320) -> (x > 0?=w322:bool)
                  n301 = case shown="真" w322 {
                    tunnel: w320 -> [_ _]
                    tunnel: w318 -> [_ w334]
                    tunnel: [w329 w330] -> w317
                    tunnel: w316 -> [w329 _]
                    frame False {
                    }
                    frame True {
                      # "最新时间戳加1分钟"
                      n302 = Array Size(array=w334) -> (size(s)=w336:i32[])
                      n303 = Index Array(array=w336) -> (element=w335:i32)  [unwired: 1 in]
                      n304 = Decrement(x=w335) -> (x-1=w333:i32)
                      n305 = Index Array(array=w334, index (row)=w333, index (col)=0 ("禁用的索引 (列)")) -> (element=w331:string)
                      n306 = call "日期时间字符串转换秒数加一.vi"("data[0]"=w331) -> ("日期/时间字符串"=w330:string)  [unwired: 10 in]
                    }
                  }
                }
                n307 = Array To Cluster(array=w312) -> (cluster=w313:T15)
                n308 = global write "全局 时间2.vi" "仪器日志索引"(w313) -> ()
              }
            }
          }
          frame #3 {
            n309 = call "数据处理整合 (子VI).vi"("枚举"=enum16{"实时数据排序", "小时数据排序"}."实时数据排序") -> ("已排序的数组"=w339:string[])  [unwired: 10 in]
            n310 = Array Size(array=w339) -> (size(s)=w338:i32)
            n311 = global write "全局 数据数组大小.vi" "数据数组大小"(w338) -> ()
          }
          frame #4 {
            # "判定是否存表"
            n312 = global read "全局 数据发送重叠.vi" "掉线指示灯"() -> (w340:bool)
            n313 = case shown="假" w340 {
              frame False {
                n314 = global read "全局 数据数组大小.vi" "数据数组大小"() -> (w341:i32)
                n315 = Greater Than 0?(x=w341) -> (x > 0?=w342:bool)
                n316 = case shown="真" w342 {
                  frame False {
                  }
                  frame True {
                    n317 = while {
                      stop <- w344 stop-if-true
                      n318 = Get Date/Time In Seconds() -> (seconds since 1Jan1904=w356:timestamp)
                      n319 = Format Date/Time String(time format string (%c)="%Y%m%d%H%M%S%3u" ("时间格式字符串(%c)"), seconds (now)=w356) -> (date/time string=w355:string)  [unwired: 1 in]
                      n320 = Search and Replace String(input string=w355, search string="." ("搜索字符串")) -> (result string=w353:string)  [unwired: 6 in, 3 out]
                      n321 = global read "断电保存全局.vi" "MN"() -> (w350:string)
                      n322 = global read "断电保存全局.vi" "PW"() -> (w349:string)
                      n323 = call "数据编码.vi"("table输入"="操作日志" ("新元素/子数组"), "QN"=w353, "MN"=w350, "PW"=w349) -> ("错误常量"=w348:errorcluster, "通讯包字符串"=w352:string)  [unwired: 10 in]
                      n324 = global read "全局 小时数据发送次数.vi" "小时数据发送次数"() -> (w345:i32)
                      n325 = global read "全局 数据数组大小.vi" "数据数组大小"() -> (w346:i32)
                      n326 = call "通信状态入队列.vi"("错误输入（无错误）"=w348, "枚举"=enum16{"打开连接", "发送数据", "读取数据", "数据处理", "关闭连接"}."发送数据") -> ()  [unwired: 9 in, 1 out]
                      n327 = global write "全局1.vi" "发送报文显示"(w352) -> ()
                      n328 = Decrement(x=w346) -> (x-1=w347:i32)
                      n329 = Greater Or Equal?(x=w345, y=w347) -> (x >= y?=w344:bool)
                      n330 = Wait (ms)(milliseconds to wait=u32 1000 ("等待时间（毫秒）")) -> ()  [unwired: 1 out]
                    }
                  }
                }
              }
              frame True {
              }
            }
          }
        }
      }
      frame "仪器参数" {
        # "间隔时间上传"
        # "直接1分钟查询 一次,有数据就按数据上传,没数据就不上传,在数据发送那边有做处理"
        n331 = flat-sequence {
          frame #0 {
            n332 = global write "全局 小时数据发送次数.vi" "小时数据发送次数"(0 ("小时数据发送次数")) -> ()
            n333 = global write "全局1.vi" "枚举"(enum16{"返回请求应答", "上传数据", "返回执行结果"}."上传数据" ("枚举")) -> ()
          }
          frame #1 {
            n334 = call "获取操作日志 (子VI).vi"("table输入"="仪器参数") -> ()  [unwired: 11 in]
          }
          frame #2 {
            n335 = global read "全局 数据发送重叠.vi" "掉线指示灯"() -> (w364:bool)
            n336 = Not(x=w364) -> (.not. x?=w363:bool)
            n337 = case shown="真" w363 {
              frame False {
              }
              frame True {
                n338 = global read "全局 时间2.vi" "仪器参数索引"() -> (w368:T16)
                n339 = Cluster To Array(cluster=w368) -> (array=w367:string[])
                n340 = for {
                  tunnel: [w372] -> w365 mode=indexing
                  tunnel: w367 -> [w371] mode=indexing
                  i -> [w370]
                  # "行数大于零"
                  n341 = case shown="12" w370 {
                    tunnel: [w376 w377 w378 w379 w380 w381 w382 w383 w384 w385 w386 w387 w388] -> w369
                    frame 0, Default {
                      n342 = global read "全局 所有参数.vi" "氨氮"() -> (w376:string[][])
                    }
                    frame 1 {
                      n343 = global read "全局 所有参数.vi" "总磷"() -> (w377:string[][])
                    }
                    frame 2 {
                      n344 = global read "全局 所有参数.vi" "总氮"() -> (w378:string[][])
                    }
                    frame 3 {
                      n345 = global read "全局 所有参数.vi" "CODMn"() -> (w379:string[][])
                    }
                    frame 4 {
                      n346 = global read "全局 所有参数.vi" "CODCr"() -> (w380:string[][])
                    }
                    frame 5 {
                      n347 = global read "全局 所有参数.vi" "DO"() -> (w381:string[][])
                    }
                    frame 6 {
                      n348 = global read "全局 所有参数.vi" "PH"() -> (w382:string[][])
                    }
                    frame 7 {
                      n349 = global read "全局 所有参数.vi" "电导率"() -> (w383:string[][])
                    }
                    frame 8 {
                      n350 = global read "全局 所有参数.vi" "水温"() -> (w384:string[][])
                    }
                    frame 9 {
                      n351 = global read "全局 所有参数.vi" "浊度"() -> (w385:string[][])
                    }
                    frame 10 {
                      n352 = global read "全局 所有参数.vi" "叶绿素"() -> (w386:string[][])
                    }
                    frame 11 {
                      n353 = global read "全局 所有参数.vi" "藻密度"() -> (w387:string[][])
                    }
                    frame 12 {
                      n354 = global read "全局 所有参数.vi" "ORP"() -> (w388:string[][])
                    }
                  }
                  n355 = Array Size(array=w369) -> (size(s)=w374:i32[])
                  n356 = Index Array(array=w374) -> (element=w373:i32)  [unwired: 1 in]
                  n357 = Greater Than 0?(x=w373) -> (x > 0?=w375:bool)
                  n358 = case shown="真" w375 {
                    tunnel: w373 -> [_ _]
                    tunnel: w369 -> [_ w393]
                    tunnel: [w389 w390] -> w372
                    tunnel: w371 -> [w389 _]
                    frame False {
                    }
                    frame True {
                      # "最新时间戳加1分钟"
                      n359 = Array Size(array=w393) -> (size(s)=w395:i32[])
                      n360 = Index Array(array=w395) -> (element=w394:i32)  [unwired: 1 in]
                      n361 = Decrement(x=w394) -> (x-1=w392:i32)
                      n362 = Index Array(array=w393, index (row)=w392, index (col)=0 ("禁用的索引 (列)")) -> (element=w396:string)
                      n363 = call "日期时间字符串转换分钟数加一.vi"("data[0]"=w396) -> ("日期/时间字符串"=w390:string)  [unwired: 10 in]
                    }
                  }
                }
                n364 = Array To Cluster(array=w365) -> (cluster=w366:T17)
                n365 = global write "全局 时间2.vi" "仪器参数索引"(w366) -> ()
              }
            }
          }
          frame #3 {
            n366 = call "数据处理整合 (子VI).vi"("枚举"=enum16{"实时数据排序", "小时数据排序"}."实时数据排序") -> ("已排序的数组"=w399:string[])  [unwired: 10 in]
            n367 = Array Size(array=w399) -> (size(s)=w398:i32)
            n368 = global write "全局 数据数组大小.vi" "数据数组大小"(w398) -> ()
          }
          frame #4 {
            # "判定是否存表"
            n369 = global read "全局 数据发送重叠.vi" "掉线指示灯"() -> (w400:bool)
            n370 = case shown="假" w400 {
              frame False {
                n371 = global read "全局 数据数组大小.vi" "数据数组大小"() -> (w401:i32)
                n372 = Greater Than 0?(x=w401) -> (x > 0?=w402:bool)
                n373 = case shown="真" w402 {
                  frame False {
                  }
                  frame True {
                    n374 = while {
                      stop <- w403 stop-if-true
                      n375 = Get Date/Time In Seconds() -> (seconds since 1Jan1904=w416:timestamp)
                      n376 = Format Date/Time String(time format string (%c)="%Y%m%d%H%M%S%3u" ("时间格式字符串(%c)"), seconds (now)=w416) -> (date/time string=w415:string)  [unwired: 1 in]
                      n377 = Search and Replace String(input string=w415, search string="." ("搜索字符串")) -> (result string=w413:string)  [unwired: 6 in, 3 out]
                      n378 = global read "断电保存全局.vi" "MN"() -> (w410:string)
                      n379 = global read "断电保存全局.vi" "PW"() -> (w409:string)
                      n380 = global read "全局 数据数组大小.vi" "数据数组大小"() -> (w405:i32)
                      n381 = call "数据编码.vi"("table输入"="仪器参数" ("新元素/子数组"), "QN"=w413, "MN"=w410, "PW"=w409) -> ("错误常量"=w408:errorcluster, "通讯包字符串"=w412:string)  [unwired: 10 in]
                      n382 = global read "全局 小时数据发送次数.vi" "小时数据发送次数"() -> (w406:i32)
                      n383 = global write "全局1.vi" "发送报文显示"(w412) -> ()
                      n384 = call "通信状态入队列.vi"("错误输入（无错误）"=w408, "枚举"=enum16{"打开连接", "发送数据", "读取数据", "数据处理", "关闭连接"}."发送数据") -> ()  [unwired: 9 in, 1 out]
                      n385 = Decrement(x=w405) -> (x-1=w404:i32)
                      n386 = Greater Or Equal?(x=w406, y=w404) -> (x >= y?=w403:bool)
                      n387 = Wait (ms)(milliseconds to wait=u32 1000 ("等待时间（毫秒）")) -> ()  [unwired: 1 out]
                    }
                  }
                }
              }
              frame True {
              }
            }
          }
        }
      }
      frame "系统状态" {
        # "直接1分钟查询 一次,有变化就按上传,没变化就不上传"
        n388 = flat-sequence {
          frame #0 {
            # "时间"
            n389 = global write "全局 小时数据发送次数.vi" "小时数据发送次数"(0 ("小时数据发送次数")) -> ()
            n390 = global write "全局 数据数组大小.vi" "数据数组大小"(1 ("数据数组大小")) -> ()
            n391 = global write "全局1.vi" "枚举"(enum16{"返回请求应答", "上传数据", "返回执行结果"}."上传数据" ("枚举")) -> ()
          }
          frame #1 {
            # "判定是否存表"
            n392 = global read "全局 数据发送重叠.vi" "掉线指示灯"() -> (w423:bool)
            n393 = case shown="假" w423 {
              frame False {
                n394 = global read "全局1.vi" "系统状态"() -> (w424:bool)
                n395 = case shown="真" w424 {
                  frame False {
                  }
                  frame True {
                    n396 = global read "全局 小时数据发送次数.vi" "小时数据发送次数"() -> (w432:i32)
                    n397 = global write "全局1.vi" "系统状态"(FALSE ("系统状态")) -> ()
                    n398 = Get Date/Time In Seconds() -> (seconds since 1Jan1904=w436:timestamp)
                    n399 = Increment(x=w432) -> (x+1=w431:i32)
                    n400 = Format Date/Time String(time format string (%c)="%Y%m%d%H%M%S%3u" ("时间格式字符串(%c)"), seconds (now)=w436) -> (date/time string=w435:string)  [unwired: 1 in]
                    n401 = global write "全局 小时数据发送次数.vi" "小时数据发送次数"(w431) -> ()
                    n402 = Search and Replace String(input string=w435, search string="." ("搜索字符串")) -> (result string=w433:string)  [unwired: 6 in, 3 out]
                    n403 = global read "断电保存全局.vi" "MN"() -> (w428:string)
                    n404 = global read "断电保存全局.vi" "PW"() -> (w427:string)
                    n405 = call "数据编码.vi"("table输入"="系统状态" ("新元素/子数组"), "QN"=w433, "MN"=w428, "PW"=w427) -> ("错误常量"=w426:errorcluster, "通讯包字符串"=w430:string)  [unwired: 10 in]
                    n406 = call "通信状态入队列.vi"("错误输入（无错误）"=w426, "枚举"=enum16{"打开连接", "发送数据", "读取数据", "数据处理", "关闭连接"}."发送数据") -> ()  [unwired: 9 in, 1 out]
                    n407 = global write "全局1.vi" "发送报文显示"(w430) -> ()
                  }
                }
              }
              frame True {
              }
            }
          }
        }
      }
      frame "运行模式" {
        # "直接1分钟查询 一次,有变化就按上传,没变化就不上传"
        n408 = flat-sequence {
          frame #0 {
            # "时间"
            n409 = global write "全局 小时数据发送次数.vi" "小时数据发送次数"(0 ("小时数据发送次数")) -> ()
            n410 = global write "全局 数据数组大小.vi" "数据数组大小"(1 ("数据数组大小")) -> ()
            n411 = global write "全局1.vi" "枚举"(enum16{"返回请求应答", "上传数据", "返回执行结果"}."上传数据" ("枚举")) -> ()
          }
          frame #1 {
            # "判定是否存表"
            n412 = global read "全局 数据发送重叠.vi" "掉线指示灯"() -> (w443:bool)
            n413 = case shown="假" w443 {
              frame False {
                n414 = global read "全局1.vi" "运行模式"() -> (w444:bool)
                n415 = case shown="真" w444 {
                  frame False {
                  }
                  frame True {
                    n416 = global read "全局 小时数据发送次数.vi" "小时数据发送次数"() -> (w452:i32)
                    n417 = global write "全局1.vi" "运行模式"(FALSE ("系统状态")) -> ()
                    n418 = Get Date/Time In Seconds() -> (seconds since 1Jan1904=w456:timestamp)
                    n419 = Increment(x=w452) -> (x+1=w451:i32)
                    n420 = Format Date/Time String(time format string (%c)="%Y%m%d%H%M%S%3u" ("时间格式字符串(%c)"), seconds (now)=w456) -> (date/time string=w455:string)  [unwired: 1 in]
                    n421 = global write "全局 小时数据发送次数.vi" "小时数据发送次数"(w451) -> ()
                    n422 = Search and Replace String(input string=w455, search string="." ("搜索字符串")) -> (result string=w453:string)  [unwired: 6 in, 3 out]
                    n423 = global read "断电保存全局.vi" "MN"() -> (w448:string)
                    n424 = global read "断电保存全局.vi" "PW"() -> (w447:string)
                    n425 = call "数据编码.vi"("table输入"="运行模式" ("新元素/子数组"), "QN"=w453, "MN"=w448, "PW"=w447) -> ("错误常量"=w446:errorcluster, "通讯包字符串"=w450:string)  [unwired: 10 in]
                    n426 = call "通信状态入队列.vi"("错误输入（无错误）"=w446, "枚举"=enum16{"打开连接", "发送数据", "读取数据", "数据处理", "关闭连接"}."发送数据") -> ()  [unwired: 9 in, 1 out]
                    n427 = global write "全局1.vi" "发送报文显示"(w450) -> ()
                  }
                }
              }
              frame True {
              }
            }
          }
        }
      }
      frame "测量周期" {
        # "直接1分钟查询 一次,有变化就按上传,没变化就不上传"
        n428 = flat-sequence {
          frame #0 {
            # "时间"
            n429 = global write "全局 小时数据发送次数.vi" "小时数据发送次数"(0 ("小时数据发送次数")) -> ()
            n430 = global write "全局 数据数组大小.vi" "数据数组大小"(1 ("数据数组大小")) -> ()
            n431 = global write "全局1.vi" "枚举"(enum16{"返回请求应答", "上传数据", "返回执行结果"}."上传数据" ("枚举")) -> ()
          }
          frame #1 {
            # "判定是否存表"
            n432 = global read "全局 数据发送重叠.vi" "掉线指示灯"() -> (w463:bool)
            n433 = case shown="假" w463 {
              frame False {
                n434 = global read "全局1.vi" "测量周期"() -> (w464:bool)
                n435 = case shown="真" w464 {
                  frame False {
                  }
                  frame True {
                    n436 = global read "全局 小时数据发送次数.vi" "小时数据发送次数"() -> (w472:i32)
                    n437 = global write "全局1.vi" "测量周期"(FALSE ("系统状态")) -> ()
                    n438 = Get Date/Time In Seconds() -> (seconds since 1Jan1904=w476:timestamp)
                    n439 = Increment(x=w472) -> (x+1=w471:i32)
                    n440 = Format Date/Time String(time format string (%c)="%Y%m%d%H%M%S%3u" ("时间格式字符串(%c)"), seconds (now)=w476) -> (date/time string=w475:string)  [unwired: 1 in]
                    n441 = global write "全局 小时数据发送次数.vi" "小时数据发送次数"(w471) -> ()
                    n442 = Search and Replace String(input string=w475, search string="." ("搜索字符串")) -> (result string=w473:string)  [unwired: 6 in, 3 out]
                    n443 = global read "断电保存全局.vi" "MN"() -> (w468:string)
                    n444 = global read "断电保存全局.vi" "PW"() -> (w467:string)
                    n445 = call "数据编码.vi"("table输入"="测量周期" ("新元素/子数组"), "QN"=w473, "MN"=w468, "PW"=w467) -> ("错误常量"=w466:errorcluster, "通讯包字符串"=w470:string)  [unwired: 10 in]
                    n446 = global write "全局1.vi" "发送报文显示"(w470) -> ()
                    n447 = call "通信状态入队列.vi"("错误输入（无错误）"=w466, "枚举"=enum16{"打开连接", "发送数据", "读取数据", "数据处理", "关闭连接"}."发送数据") -> ()  [unwired: 9 in, 1 out]
                  }
                }
              }
              frame True {
              }
            }
          }
        }
      }
      frame "超标留样" {
        # "直接1分钟查询 一次,有变化就按上传,没变化就不上传"
        n448 = flat-sequence {
          frame #0 {
            # "时间"
            n449 = global write "全局 小时数据发送次数.vi" "小时数据发送次数"(0 ("小时数据发送次数")) -> ()
            n450 = global write "全局 数据数组大小.vi" "数据数组大小"(1 ("数据数组大小")) -> ()
            n451 = global write "全局1.vi" "枚举"(enum16{"返回请求应答", "上传数据", "返回执行结果"}."上传数据" ("枚举")) -> ()
          }
          frame #1 {
            # "判定是否存表"
            n452 = global read "全局 数据发送重叠.vi" "掉线指示灯"() -> (w483:bool)
            n453 = case shown="假" w483 {
              frame False {
                n454 = global read "全局1.vi" "超标留样"() -> (w484:bool)
                n455 = case shown="真" w484 {
                  frame False {
                  }
                  frame True {
                    n456 = global read "全局 小时数据发送次数.vi" "小时数据发送次数"() -> (w492:i32)
                    n457 = global write "全局1.vi" "超标留样"(FALSE ("系统状态")) -> ()
                    n458 = Get Date/Time In Seconds() -> (seconds since 1Jan1904=w496:timestamp)
                    n459 = Increment(x=w492) -> (x+1=w491:i32)
                    n460 = Format Date/Time String(time format string (%c)="%Y%m%d%H%M%S%3u" ("时间格式字符串(%c)"), seconds (now)=w496) -> (date/time string=w495:string)  [unwired: 1 in]
                    n461 = global write "全局 小时数据发送次数.vi" "小时数据发送次数"(w491) -> ()
                    n462 = Search and Replace String(input string=w495, search string="." ("搜索字符串")) -> (result string=w493:string)  [unwired: 6 in, 3 out]
                    n463 = global read "断电保存全局.vi" "MN"() -> (w487:string)
                    n464 = global read "断电保存全局.vi" "PW"() -> (w486:string)
                    n465 = call "数据编码.vi"("table输入"="超标留样" ("新元素/子数组"), "QN"=w493, "MN"=w487, "PW"=w486) -> ("错误常量"=w488:errorcluster, "通讯包字符串"=w490:string)  [unwired: 10 in]
                    n466 = global write "全局1.vi" "发送报文显示"(w490) -> ()
                    n467 = call "通信状态入队列.vi"("错误输入（无错误）"=w488, "枚举"=enum16{"打开连接", "发送数据", "读取数据", "数据处理", "关闭连接"}."发送数据") -> ()  [unwired: 9 in, 1 out]
                  }
                }
              }
              frame True {
              }
            }
          }
        }
      }
      frame "报警信息" {
        # "间隔时间上传"
        # "直接1分钟查询 一次,有数据就按数据上传,没数据为空的不传,在数据发送那边有做处理"
        n468 = flat-sequence {
          frame #0 {
            # "分钟时间间隔"
            n469 = call "日志信息主动发送(子VI).vi"() -> ()  [unwired: 12 in]
            n470 = global write "全局 小时数据发送次数.vi" "小时数据发送次数"(0 ("小时数据发送次数")) -> ()
            n471 = global write "全局1.vi" "枚举"(enum16{"返回请求应答", "上传数据", "返回执行结果"}."上传数据" ("枚举")) -> ()
          }
          frame #1 {
            n472 = call "获取报警信息 (子VI).vi"() -> ()  [unwired: 12 in]
          }
          frame #2 {
            n473 = global read "全局 数据发送重叠.vi" "掉线指示灯"() -> (w503:bool)
            n474 = Not(x=w503) -> (.not. x?=w502:bool)
            n475 = case shown="真" w502 {
              frame False {
              }
              frame True {
                n476 = global read "全局 时间2.vi" "报警信息索引"() -> (w507:T18)
                n477 = Cluster To Array(cluster=w507) -> (array=w506:string[])
                n478 = for {
                  tunnel: [w509] -> w504 mode=indexing
                  tunnel: w506 -> [w508] mode=indexing
                  i -> [w511]
                  # "行数大于零"
                  n479 = case shown="1" w511 {
                    tunnel: [w515 w516 w517 w518 w519 w520 w521 w522 w523 w524 w525 w526] -> w510
                    frame 0, Default {
                      n480 = global read "全局 所有参数.vi" "氨氮"() -> (w515:string[][])
                    }
                    frame 1 {
                      n481 = global read "全局 所有参数.vi" "总磷"() -> (w516:string[][])
                    }
                    frame 2 {
                      n482 = global read "全局 所有参数.vi" "总氮"() -> (w517:string[][])
                    }
                    frame 3 {
                      n483 = global read "全局 所有参数.vi" "CODMn"() -> (w518:string[][])
                    }
                    frame 4 {
                      n484 = global read "全局 所有参数.vi" "CODCr"() -> (w519:string[][])
                    }
                    frame 5 {
                      n485 = global read "全局 所有参数.vi" "DO"() -> (w520:string[][])
                    }
                    frame 6 {
                      n486 = global read "全局 所有参数.vi" "PH"() -> (w521:string[][])
                    }
                    frame 7 {
                      n487 = global read "全局 所有参数.vi" "电导率"() -> (w522:string[][])
                    }
                    frame 8 {
                      n488 = global read "全局 所有参数.vi" "水温"() -> (w523:string[][])
                    }
                    frame 9 {
                      n489 = global read "全局 所有参数.vi" "浊度"() -> (w524:string[][])
                    }
                    frame 10 {
                      n490 = global read "全局 所有参数.vi" "叶绿素"() -> (w525:string[][])
                    }
                    frame 11 {
                      n491 = global read "全局 所有参数.vi" "藻密度"() -> (w526:string[][])
                    }
                  }
                  n492 = Array Size(array=w510) -> (size(s)=w513:i32[])
                  n493 = Index Array(array=w513) -> (element=w512:i32)  [unwired: 1 in]
                  n494 = Greater Than 0?(x=w512) -> (x > 0?=w514:bool)
                  n495 = case shown="真" w514 {
                    tunnel: w512 -> [_ _]
                    tunnel: w510 -> [_ w531]
                    tunnel: [w527 w528] -> w509
                    tunnel: w508 -> [w527 _]
                    frame False {
                    }
                    frame True {
                      # "最新时间戳加1分钟"
                      n496 = Array Size(array=w531) -> (size(s)=w533:i32[])
                      n497 = Index Array(array=w533) -> (element=w532:i32)  [unwired: 1 in]
                      n498 = Decrement(x=w532) -> (x-1=w530:i32)
                      n499 = Index Array(array=w531, index (row)=w530, index (col)=0 ("禁用的索引 (列)")) -> (element=w534:string)
                      n500 = call "日期时间字符串转换分钟数加一.vi"("data[0]"=w534) -> ("日期/时间字符串"=w528:string)  [unwired: 10 in]
                    }
                  }
                }
                n501 = Array To Cluster(array=w504) -> (cluster=w505:T19)
                n502 = global write "全局 时间2.vi" "报警信息索引"(w505) -> ()
              }
            }
          }
          frame #3 {
            n503 = call "数据处理整合 (子VI).vi"("枚举"=enum16{"实时数据排序", "小时数据排序"}."实时数据排序") -> ("已排序的数组"=w537:string[])  [unwired: 10 in]
            n504 = Array Size(array=w537) -> (size(s)=w536:i32)
            n505 = global write "全局 数据数组大小.vi" "数据数组大小"(w536) -> ()
          }
          frame #4 {
            # "判定是否存表"
            n506 = global read "全局 数据发送重叠.vi" "掉线指示灯"() -> (w538:bool)
            n507 = case shown="假" w538 {
              frame False {
                # "判定数据不为空才发"
                n508 = global read "全局 数据数组大小.vi" "数据数组大小"() -> (w539:i32)
                n509 = Greater Than 0?(x=w539) -> (x > 0?=w540:bool)
                n510 = case shown="真" w540 {
                  frame False {
                    n511 = global write "全局1.vi" "核查数据上传"(FALSE ("数据上传")) -> ()
                  }
                  frame True {
                    n512 = while {
                      stop <- w543 stop-if-true
                      n513 = Wait (ms)(milliseconds to wait=u32 1000 ("等待时间（毫秒）")) -> ()  [unwired: 1 out]
                      n514 = Get Date/Time In Seconds() -> (seconds since 1Jan1904=w555:timestamp)
                      n515 = Format Date/Time String(time format string (%c)="%Y%m%d%H%M%S%3u" ("时间格式字符串(%c)"), seconds (now)=w555) -> (date/time string=w554:string)  [unwired: 1 in]
                      n516 = global read "全局 数据数组大小.vi" "数据数组大小"() -> (w545:i32)
                      n517 = Search and Replace String(input string=w554, search string="." ("搜索字符串")) -> (result string=w552:string)  [unwired: 6 in, 3 out]
                      n518 = global read "断电保存全局.vi" "MN"() -> (w549:string)
                      n519 = global read "断电保存全局.vi" "PW"() -> (w548:string)
                      n520 = global read "全局 小时数据发送次数.vi" "小时数据发送次数"() -> (w546:i32)
                      n521 = call "数据编码.vi"("table输入"="报警信息" ("新元素/子数组"), "QN"=w552, "MN"=w549, "PW"=w548) -> ("错误常量"=w547:errorcluster, "通讯包字符串"=w551:string)  [unwired: 10 in]
                      n522 = Decrement(x=w545) -> (x-1=w544:i32)
                      n523 = global write "全局1.vi" "发送报文显示"(w551) -> ()
                      n524 = Greater Or Equal?(x=w546, y=w544) -> (x >= y?=w543:bool)
                      n525 = call "通信状态入队列.vi"("错误输入（无错误）"=w547, "枚举"=enum16{"打开连接", "发送数据", "读取数据", "数据处理", "关闭连接"}."发送数据") -> ()  [unwired: 9 in, 1 out]
                    }
                  }
                }
              }
              frame True {
              }
            }
          }
        }
      }
      frame "环境参数" {
        n526 = call "核查数据断电保存 (子VI).vi"() -> ()  [unwired: 12 in]
      }
    }
    n527 = Not(x=w4) -> (.not. x?=w5:bool)
    n528 = global write "全局1.vi" "核查数据上传"(w5) -> ()
  }
  "错误输出" <- w1
